vi "FileMan Print File.vi"(0 "error in (no error)":errorcluster, 1 "show (1:Normal)":i16(ring)=1 items=["SW_HIDE", "SW_SHOWNORMAL", "SW_SHOWMINIMIZED"], 5 "path to file (empty path)":path) -> (3 "error out":errorcluster)   [LabVIEW 2011]
doc: "This VI will print a file whose extension is associated with an application, as available in Windows' File Manager. For example, files with the .wri extension are usually associated with the Windows application Write. A file with the extension .wri will then be printed using Microsoft Write.\n\nFiles whose extensions are not associated with an application, or applications which do not support file printing from the File Manager, will return an error."
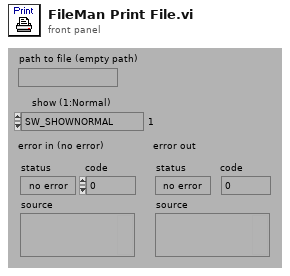
[diagram p1: front panel]
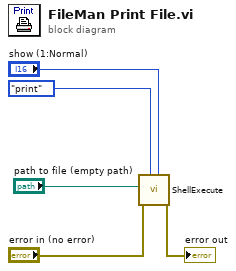
[diagram p0: block diagram]
diagram:
  n1 = call "ShellExecute.vi"("show"="show (1:Normal)", "operation (open)"=enum16{"open", "print"}."print", "error in (no error)"="error in (no error)", "path to file"="path to file (empty path)") -> ("error out"=→"error out":errorcluster)  [unwired: 3 in, 4 out]
